vi "Grid KeyDown RingCol.vi"(4 "表サイズ(縦×横)":i32[](array[numeric]), 6 "EditPos":T1, 8 "エラー入力（エラーなし）":errorcluster, 9 "Char":i16, 10 "ref.表":refnum<vi>, 11 "Control入力":refnum<vi>) -> (0 "error out":errorcluster caption="エラー出力", 1 "セル文字列":string, 3 "破棄?":bool)   [LabVIEW 2014]
uses:
  <vilib>/event_ctls.llb/eventvkey.ctl
  <vilib>/Utility/miscctls.llb/LVRowAndColumnTypeDef.ctl
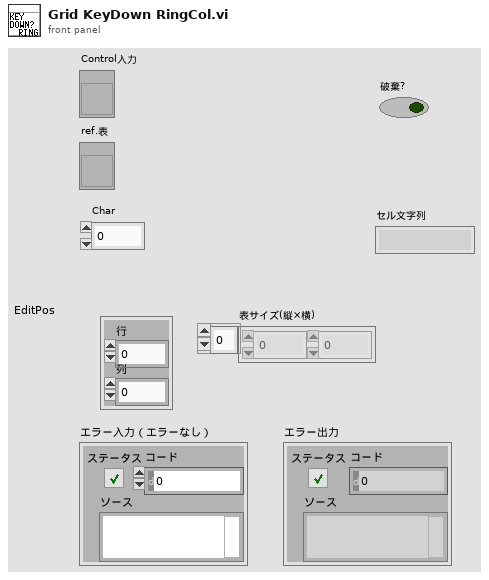
[diagram p1: front panel]
types:
  T1 = typedef "LVRowAndColumnTypeDef.ctl" = cluster{"Row":i32, "Column":i32}
  T2 = typedef "eventvkey.ctl" = enum16{"ASCII", "Enter", "Return", "Shift", "Ctrl", "Alt", "Cmd", "Opt", "Caps", "NumLock", "Clear", "Break", "Up", "Down", "Left", "Right", "Insert", "Delete", "Home", "End", "PageUp", "PageDown", "Escape", "Help", "Pause", "ScrollLock", "F1", "F2", "F3", "F4", "F5", "F6", "F7", "F8", "F9", "F10", "F11", "F12", "F13", "F14", "F15", "F16", "F17", "F18", "F19", "F20", "F21", "F22", "F23", "F24", "Play", "VolumeUp", "VolumeDown", "Mute", "Two Byte Char"}
  T3 = typedef "LVStringsAndValuesArrayTypeDef.ctl" = cluster{"String":string, "Value":ext}[]
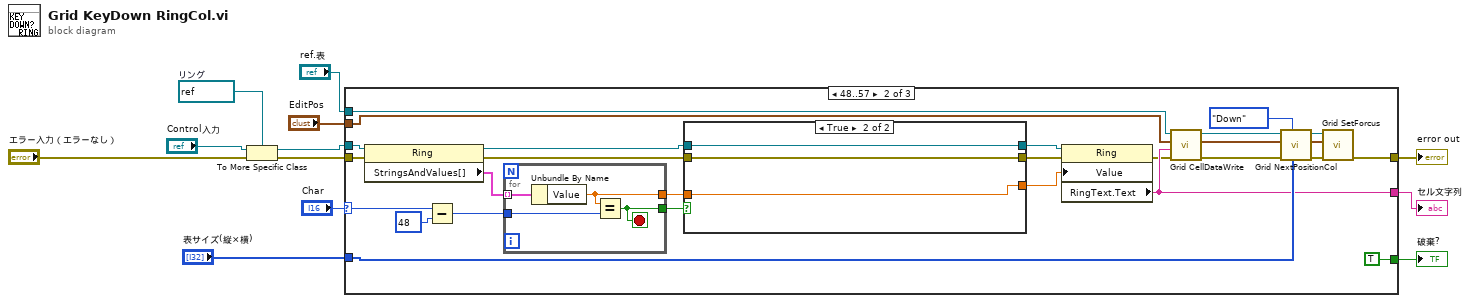
[diagram p0: block diagram]
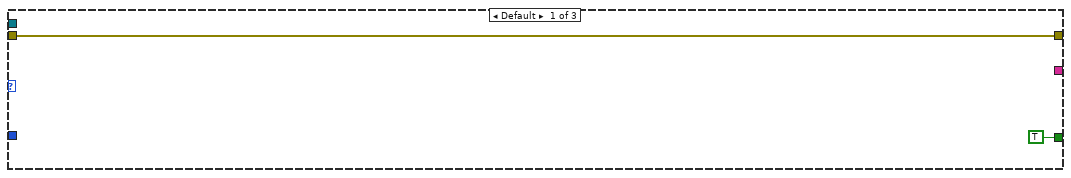
[diagram p2: hidden frame]
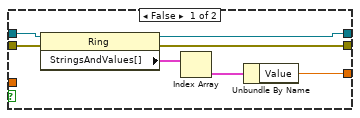
[diagram p3: hidden frame]
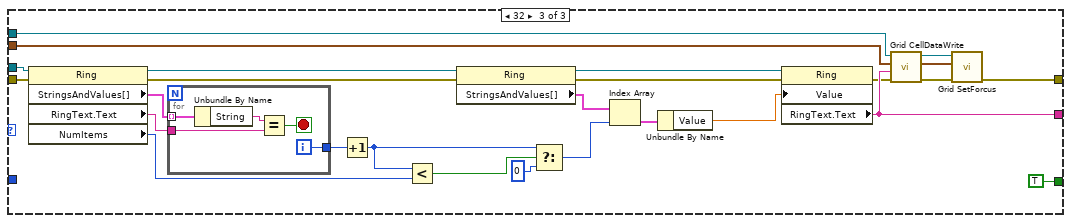
[diagram p4: hidden frame]
diagram:
  w7 = refnum<vi> refnum  # リング
  n1 = To More Specific Class(target class=w7, reference="Control入力", error in="エラー入力（エラーなし）") -> (specific class reference=w9:refnum<vi>, error out=w1:errorcluster)
  n2 = case shown="48..57" "Char" {
    selector: "Char" -> [_ w40 _]
    tunnel: "EditPos" -> [_ w33 w78]
    tunnel: "表サイズ(縦×横)" -> [_ w37 _]
    tunnel: w9 -> [_ w36 w80]
    tunnel: "ref.表" -> [_ w34 w79]
    tunnel: [TRUE TRUE TRUE] -> w11
    tunnel: [w13 w20 w67] -> w3
    tunnel: [_ w21 w66] -> w2
    tunnel: w1 -> [w13 w19 w65]
    frame Default {
    }
    frame 48..57 {
      n3 = property class="Ring"(reference=w36, error in=w19) -> (reference out=w26:refnum<vi>, error out=w18:errorcluster, "StringsAndValues[]"=w39:T3)
      n4 = Subtract(x=w40, y=48) -> (x-y=w38:i32)
      n5 = for {
        tunnel: w39 -> [w53] mode=indexing
        tunnel: w38 -> [w55]
        tunnel: [w54] -> w29
        tunnel: [w52] -> w27
        stop <- w54 stop-if-true
        n6 = Unbundle By Name(w53) -> ("Value"=w52:ext)
        n7 = Equal?(x=w52, y=w55) -> (x = y?=w54:bool)
      }
      n8 = case shown="TRUE" w29 {
        tunnel: [w45 w51] -> w28
        tunnel: w27 -> [_ w51]
        tunnel: w26 -> [w48 w50]
        tunnel: w18 -> [w44 w49]
        tunnel: [w43 w50] -> w17
        tunnel: [w42 w49] -> w16
        frame False {
          n9 = property class="Ring"(reference=w48, error in=w44) -> (reference out=w43:refnum<vi>, error out=w42:errorcluster, "StringsAndValues[]"=w47:T3)
          n10 = Index Array(array=w47) -> (element=w46:cluster{"String":string, "Value":ext})  [unwired: 1 in]
          n11 = Unbundle By Name(w46) -> ("Value"=w45:ext)
        }
        frame True {
        }
      }
      n12 = property class="Ring"(reference=w17, error in=w16, "Value"=w28) -> (error out=w15:errorcluster, "RingText.Text"=w21:string)  [unwired: 1 out]
      n13 = call "Grid CellDataWrite.vi"("error in (no error)"=w15, "RingText.Text"=w21, "EditPos"=w33, "Table入力"=w34) -> ("エラー出力"=w30:errorcluster, "EditPos(copy))"=w31:T1, "Table出力"=w32:refnum<vi>)  [unwired: 5 in]
      n14 = call "Grid NextPositionCol.vi"("表サイズ(縦x横)"=w37, "VKey(Right)"=eventvkey."Down" ("VKey"), "error in (no error)"=w30, "EditPos入力"=w31, "ref.表"=w32) -> ("error out"=w23:errorcluster, "EditPos出力"=w24:T1, "ref.表(copy)"=w25:refnum<vi>)  [unwired: 4 in]
      n15 = call "Grid SetForcus.vi"("エラー入力（エラーなし）"=w23, "EditPos入力"=w24, "Table入力"=w25) -> ("error out"=w20:errorcluster)  [unwired: 6 in, 2 out]
    }
    frame 32 {
      n16 = property class="Ring"(reference=w80, error in=w65) -> (reference out=w63:refnum<vi>, error out=w61:errorcluster, "StringsAndValues[]"=w81:T3, "RingText.Text"=w77:string, "NumItems"=w75:u32)
      n17 = for {
        tunnel: w81 -> [w85] mode=indexing
        tunnel: w77 -> [w83]
        tunnel: [w82] -> w76
        i -> [w82]
        stop <- w86 stop-if-true
        n18 = Unbundle By Name(w85) -> ("String"=w84:string)
        n19 = Equal?(x=w84, y=w83) -> (x = y?=w86:bool)
      }
      n20 = Increment(x=w76) -> (x+1=w72:i32)
      n21 = Less?(x=w72, y=w75) -> (x < y?=w74:bool)
      n22 = property class="Ring"(reference=w63, error in=w61) -> (reference out=w62:refnum<vi>, error out=w60:errorcluster, "StringsAndValues[]"=w59:T3)
      n23 = Select(t=w72, s=w74, f=0 ("t")) -> (s? t:f=w58:i32)
      n24 = Index Array(array=w59, index=w58) -> (element=w57:cluster{"String":string, "Value":ext})
      n25 = Unbundle By Name(w57) -> ("Value"=w56:ext)
      n26 = property class="Ring"(reference=w62, error in=w60, "Value"=w56) -> (error out=w64:errorcluster, "RingText.Text"=w66:string)  [unwired: 1 out]
      n27 = call "Grid CellDataWrite.vi"("error in (no error)"=w64, "RingText.Text"=w66, "EditPos"=w78, "Table入力"=w79) -> ("エラー出力"=w68:errorcluster, "EditPos(copy))"=w70:T1, "Table出力"=w69:refnum<vi>)  [unwired: 5 in]
      n28 = call "Grid SetForcus.vi"("エラー入力（エラーなし）"=w68, "EditPos入力"=w70, "Table入力"=w69) -> ("error out"=w67:errorcluster)  [unwired: 6 in, 2 out]
    }
  }
  "破棄?" <- w11
  "error out" <- w3
  "セル文字列" <- w2
